vi "testOfcClasses.vi"(8 "error in (no error)":errorcluster) -> (0 "error out":errorcluster)   [LabVIEW 2016]
doc: "Test all OFC classes."
uses:
  <vilib>/addons/_JKI Toolkits/Caraya/classes/Test/Test.lvclass
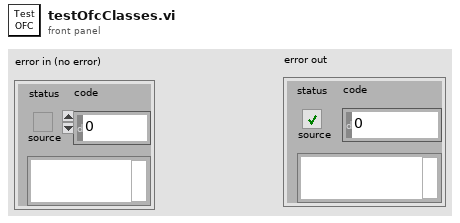
[diagram p1: front panel]
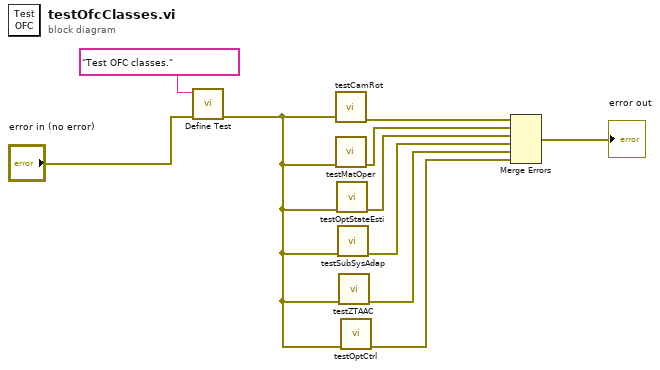
[diagram p0: block diagram]
diagram:
  n1 = call <vilib>:"Define Test.vi"("error in (no error)"="error in (no error)", "Label (VI Title)"="Test OFC classes.") -> ("error out"=w8:errorcluster)  [unwired: 9 in]
  n2 = call "testCamRot.vi"("error in (no error)"=w8) -> ("error out"=w7:errorcluster)  [unwired: 10 in]
  n3 = call "testMatOper.vi"("error in (no error)"=w8) -> ("error out"=w6:errorcluster)  [unwired: 10 in]
  n4 = call "testOptStateEsti.vi"("error in (no error)"=w8) -> ("error out"=w5:errorcluster)  [unwired: 10 in]
  n5 = call "testSubSysAdap.vi"("error in (no error)"=w8) -> ("error out"=w4:errorcluster)  [unwired: 10 in]
  n6 = call "testZTAAC.vi"("error in (no error)"=w8) -> ("error out"=w3:errorcluster)  [unwired: 10 in]
  n7 = call "testOptCtrl.vi"("error in (no error)"=w8) -> ("error out"=w2:errorcluster)  [unwired: 10 in]
  n8 = Merge Errors(w7, w6, w5, w4, w3, w2) -> (→"error out":errorcluster)
